vi "Configure IQ vs Slot Measurement Parameters.vi"(6 "Frequency Error Limit (-100Hz)":dbl=-100.0 format="%#.9p", 7 "Step Length (1.0E-3)":dbl=0.001 format="%#_6f", 8 "error in (no error)":errorcluster, 9 "Measurement Length (0.0008)":dbl=0.0008, 10 "Instance (1)":i32=1 format="%.0g", 11 "VISA resource name":refnum<visa-resource-name>) -> (0 "error out":errorcluster, 3 "VISA resource name out":refnum<visa-resource-name>)   [LabVIEW 2015, in "Rohde&Schwarz CMXP GPRF.lvlib"]
doc: "Configures IQ vs Slot measurement parameters.\n\nAttributes:\nRSCMXPGPRF_ATTR_IQ_VS_SLOT_MEASUREMENT_MEASUREMENT_LENGTH\nRSCMXPGPRF_ATTR_IQ_VS_SLOT_MEASUREMENT_STEP_LENGTH\nRSCMXPGPRF_ATTR_IQ_VS_SLOT_MEASUREMENT_FREQUENCY_ERROR_LIMIT\n\nRemote-control commands:\nCONFigure:GPRF:MEAS<i>:IQVSlot:MLENgth\nCONFigure:GPRF:MEAS<i>:IQVSlot:SLENgth\nCONFigure:GPRF:MEAS<i>:IQVSlot:FELimit"
uses:
  <instrlib>/Rohde&Schwarz CMXP GPRF/Rohde&Schwarz CMXP GPRF.lvlib
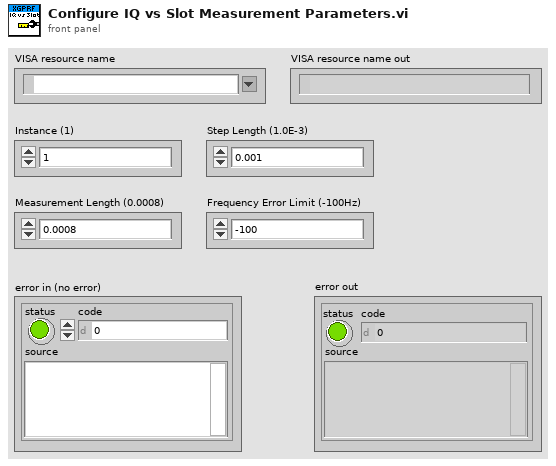
[diagram p1: front panel]
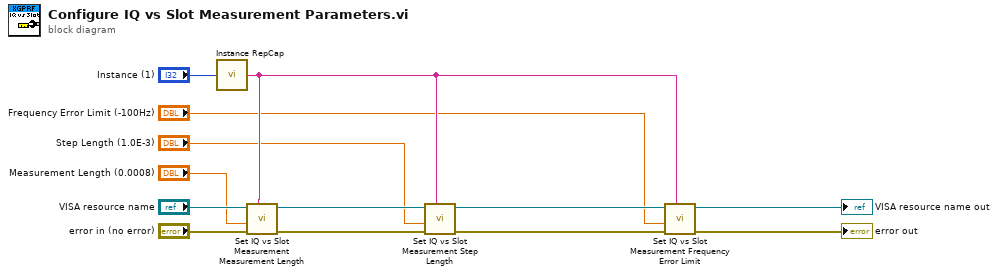
[diagram p0: block diagram]
diagram:
  n1 = call <instrlib>:"Instance RepCap.vi"("instance  in"="Instance (1)") -> ("instance out"=w6:string)
  n2 = call "Set IQ vs Slot Measurement Measurement Length"("Repeated Capabilities"=w6, "error in (no error)"="error in (no error)", "IQ vs Slot Measurement Measurement Length (0.0)"="Measurement Length (0.0008)", "instrument handle"="VISA resource name") -> ("error out"=w11:errorcluster, "instrument handle out"=w12:refnum<visa-resource-name>)  [unwired: 6 in]
  n3 = call "Set IQ vs Slot Measurement Step Length"("Repeated Capabilities"=w6, "error in (no error)"=w11, "IQ vs Slot Measurement Step Length (0.0)"="Step Length (1.0E-3)", "instrument handle"=w12) -> ("error out"=w9:errorcluster, "instrument handle out"=w10:refnum<visa-resource-name>)  [unwired: 6 in]
  n4 = call "Set IQ vs Slot Measurement Frequency Error Limit"("Repeated Capabilities"=w6, "error in (no error)"=w9, "IQ vs Slot Measurement Frequency Error Limit (0.0)"="Frequency Error Limit (-100Hz)", "instrument handle"=w10) -> ("error out"=→"error out":errorcluster, "instrument handle out"=→"VISA resource name out":refnum<visa-resource-name>)  [unwired: 6 in]
